vi "Wiimote LEDs Write.vi"(8 "error in (no error)":errorcluster, 9 "Wiimote Player #":i32=1, 10 "Wiimote LEDs In":T1, 11 "LV WiiMote Interface In":T2) -> (0 "error out":errorcluster, 2 "Wiimote LEDs out":T1, 3 "LV WiiMote Interface out":T2)   [LabVIEW 2012, in "LV Wiimote Interface.lvclass"]
uses:
  LV Wiimote Interface.lvclass
  Controls/LV Wiimote Interface.ctl
  Controls/Wiimote LEDs.ctl
  C:/Program Files/National Instruments/LabVIEW 2012/vi.lib/LabVIEW Hacker/WiiMote/Dependencies/WiimoteLib.dll
  Program Files/National Instruments/LabVIEW 2012/vi.lib/LabVIEW Hacker/WiiMote/Dependencies/WiimoteLib.dll
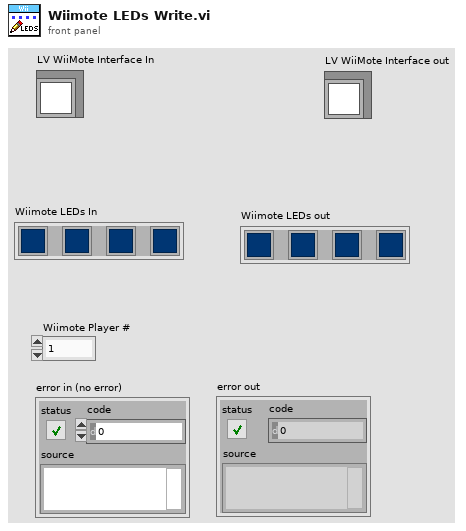
[diagram p1: front panel]
types:
  T1 = typedef "LV Wiimote Interface.lvclass/Wiimote LEDs.ctl" = cluster{"Wiimote LED":bool, "Wiimote LED 2":bool, "Wiimote LED 3":bool, "Wiimote LED 4":bool}
  T2 = typedef "LV Wiimote Interface.ctl" = refnum<class "LV Wiimote Interface.lvclass">
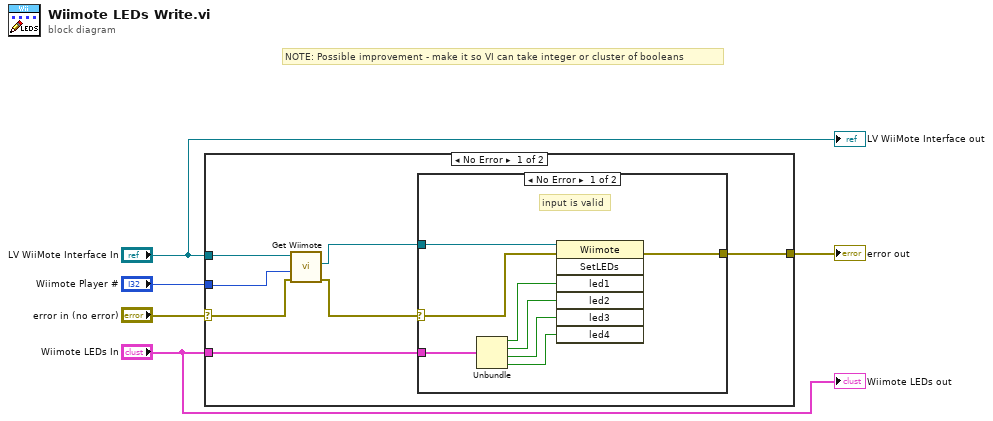
[diagram p0: block diagram]
diagram:
  # "NOTE: Possible improvement - make it so VI can take integer or cluster of booleans"
  n1 = case shown="No Error" "error in (no error)" {
    selector: "error in (no error)" -> [w9 w22]
    tunnel: "LV WiiMote Interface In" -> [w11 _]
    tunnel: "Wiimote LEDs In" -> [w12 _]
    tunnel: "Wiimote Player #" -> [w10 _]
    tunnel: [w6 w22] -> w3
    frame No Error {
      n2 = call "Get Wiimote.vi"("error in (no error)"=w9, "Wiimote Player #"=w10, "LV Wiimote Interface in"=w11) -> ("error out"=w8:errorcluster, "Wiimote"=w7:refnum<k24>)  [unwired: 6 in, 1 out]
      n3 = case shown="No Error" w8 {
        selector: w8 -> [w15 w21]
        tunnel: w12 -> [w20 _]
        tunnel: [w14 w21] -> w6
        tunnel: w7 -> [w13 _]
        frame No Error {
          # "input is valid"
          n4 = Unbundle(w20) -> ("Wiimote LED"=w19:bool, "Wiimote LED 2"=w18:bool, "Wiimote LED 3"=w17:bool, "Wiimote LED 4"=w16:bool)
          n5 = invoke class="Wiimote" method="SetLEDs"(reference=w13, error in=w15, "led1"=w19, "led2"=w18, "led3"=w17, "led4"=w16) -> (error out=w14:errorcluster)  [unwired: 1 in, 6 out]
        }
        frame Error {
          # "Selected Wiimote # larger than \nnumber of Wiimotes available"
        }
      }
    }
    frame Error {
    }
  }
  "error out" <- w3
  "LV WiiMote Interface out" <- "LV WiiMote Interface In"
  "Wiimote LEDs out" <- "Wiimote LEDs In"
